vi "Append Keyword.vi"(0 "Display State In":T1, 5 "New Keyword":string, 9 "Container State":T2, 11 "error in (no error)":errorcluster) -> (4 "Display State Out":T1, 15 "error out":errorcluster)   [LabVIEW 2011, in "Intellisense Xcontrol.xctl"]
uses:
  Intellisense Xcontrol.xctl
  <vilib>/_xctls/Container State.ctl
  State 1.ctl
  <vilib>/_xctls/XControlSupport.lvlib
panel:
  # "Add Controls & Indicators that form the parameters of the method here. Hook them to the connector pane. Do not delete the controls & indicators that are already hooked to the connector pane.\n \nTo setup the parameters  for this method, right click on this item in the Project Tree & select \"Configure Method...\"."
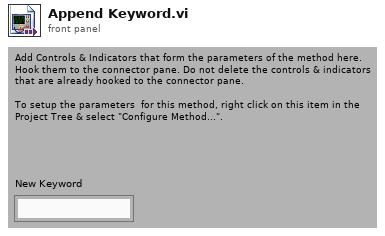
[diagram p1: front panel]
types:
  T1 = typedef "Intellisense Xcontrol.xctl/State 1.ctl" = cluster{"Keyword Array":string[], "Auto-Complete On/Off":bool, "Delimiter":string, "error in (no error)":errorcluster}
  T2 = typedef "XControlSupport.lvlib/Container State.ctl" = cluster{"Indicator?":bool, "Run Mode?":bool, " Refnum":refnum<vi>}
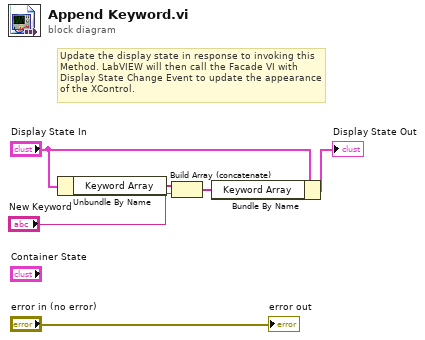
[diagram p0: block diagram]
diagram:
  # "Update the display state in response to invoking this Method. LabVIEW will then call the Facade VI with Display State Change Event to update the appearance of the XControl."
  n1 = Unbundle By Name("Display State In") -> ("Keyword Array"=w5:string[])
  n2 = Build Array (concatenate)(w5, "New Keyword") -> (w2:string[])
  n3 = Bundle By Name(cluster="Display State In", "Keyword Array"=w2) -> (→"Display State Out":T1)
  "error out" <- "error in (no error)"
